vi "Queue Driver.vi"(0 "Queue Name":string, 2 "State[]":cluster{"State":string, "Data":variant}[](array[cluster]), 11 "Error In":errorcluster, 13 "Q Operations":T1(ring)) -> (4 "Dequeued State":cluster{"State":string, "Data":variant}, 15 "Error Out":errorcluster)   [LabVIEW 2020]
doc: "This is the queue driver VI. Which works like an LV2. It stores the queue refnum in the shift register to perform the queue operation based on the selected option in the Q Operation enum"
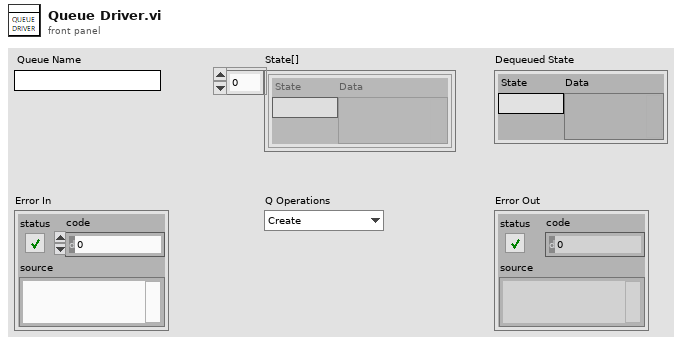
[diagram p1: front panel]
types:
  T1 = enum16{"Create", "Enqueue", "Dequeue", "Enstack", "Flush", "Destroy"}
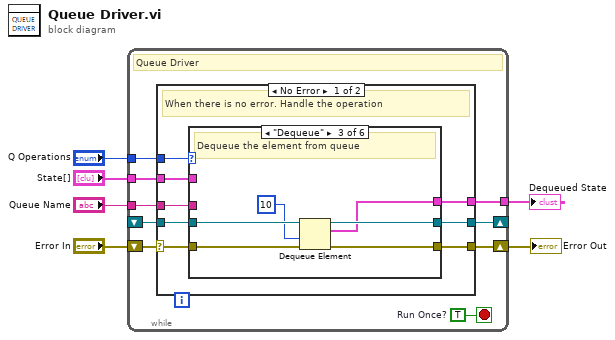
[diagram p0: block diagram]
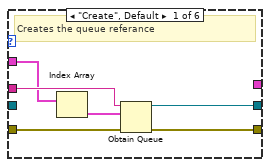
[diagram p2: hidden frame]
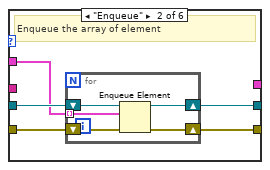
[diagram p3: hidden frame]
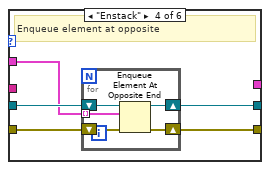
[diagram p4: hidden frame]
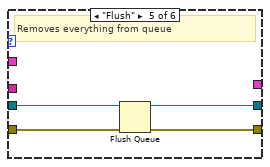
[diagram p5: hidden frame]
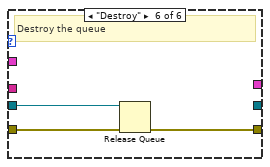
[diagram p6: hidden frame]
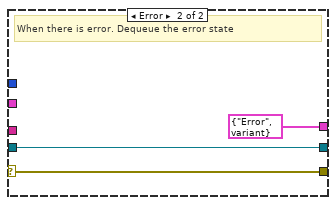
[diagram p7: hidden frame]
diagram:
  n1 = while {
    shift-right: [w13] -> w1
    shift-left: "Error In" -> [w14]
    tunnel: "Queue Name" -> [w12]
    shift-right: [w11] -> _
    shift-left: _ -> [w10]
    tunnel: "Q Operations" -> [w9]
    tunnel: "State[]" -> [w8]
    tunnel: [w7] -> w2
    stop <- w15 stop-if-true
    w15 = TRUE  # Run Once?
    # "Queue Driver"
    n2 = case shown="No Error" w14 {
      selector: w14 -> [w23 w64]
      tunnel: [w22 w64] -> w13
      tunnel: w12 -> [w21 _]
      tunnel: [w20 w65] -> w11
      tunnel: w10 -> [w18 w65]
      tunnel: w9 -> [w19 _]
      tunnel: w8 -> [w17 _]
      tunnel: [w16 cluster{"State":string, "Data":variant} {"State"="Error", "Data"=variant} ("State")] -> w7
      frame No Error {
        # "When there is no error. Handle the operation"
        n3 = case shown="\"Dequeue\"" w19 {
          tunnel: w23 -> [w29 w34 w45 w50 w59 w62]
          tunnel: [w28 w33 w44 w49 w58 w61] -> w22
          tunnel: w21 -> [w27 _ _ _ _ _]
          tunnel: [w26 w31 w42 w47 w56 _] -> w20
          tunnel: w18 -> [_ w32 w43 w48 w57 w60]
          tunnel: w17 -> [w25 w30 _ w46 _ _]
          tunnel: [_ _ w41 _ _ _] -> w16
          frame "Create", Default {
            # "Creates the queue referance"
            n4 = Index Array(array=w25) -> (element=w24:cluster{"State":string, "Data":variant})  [unwired: 1 in]
            n5 = Obtain Queue(name (unnamed)=w27, element data type=w24, error in (no error)=w29) -> (queue out=w26:refnum<queue>, error out=w28:errorcluster)  [unwired: 2 in, 1 out]
          }
          frame "Enqueue" {
            # "Enqueue the array of element"
            n6 = for {
              tunnel: w30 -> [w35] mode=indexing
              shift-right: [w38] -> w33
              shift-left: w34 -> [w39]
              shift-right: [w36] -> w31
              shift-left: w32 -> [w37]
              n7 = Enqueue Element(queue=w37, element=w35, error in (no error)=w39) -> (queue out=w36:refnum<queue>, error out=w38:errorcluster)  [unwired: 1 in, 1 out]
            }
          }
          frame "Dequeue" {
            # "Dequeue the element from queue"
            n8 = Dequeue Element(queue=w43, timeout in ms (-1)=10, error in (no error)=w45) -> (queue out=w42:refnum<queue>, element=w41:cluster{"State":string, "Data":variant}, error out=w44:errorcluster)  [unwired: 1 out]
          }
          frame "Enstack" {
            # "Enqueue element at opposite"
            n9 = for {
              tunnel: w46 -> [w51] mode=indexing
              shift-right: [w54] -> w49
              shift-left: w50 -> [w55]
              shift-right: [w52] -> w47
              shift-left: w48 -> [w53]
              n10 = Enqueue Element At Opposite End(queue=w53, element=w51, error in (no error)=w55) -> (queue out=w52:refnum<queue>, error out=w54:errorcluster)  [unwired: 1 in, 1 out]
            }
          }
          frame "Flush" {
            # "Removes everything from queue"
            n11 = Flush Queue(queue=w57, error in (no error)=w59) -> (queue out=w56:refnum<queue>, error out=w58:errorcluster)  [unwired: 1 out]
          }
          frame "Destroy" {
            # "Destroy the queue"
            n12 = Release Queue(queue=w60, error in (no error)=w62) -> (error out=w61:errorcluster)  [unwired: 1 in, 2 out]
          }
        }
      }
      frame Error {
        # "When there is error. Dequeue the error state"
      }
    }
  }
  "Error Out" <- w1
  "Dequeued State" <- w2
